vi "Offset_decoder_CH0_no_sign.vi"(11 "Array In1":i8[](array[numeric])) -> (3 "CH0":i32)   [LabVIEW 2012]
panel:
  out "CH0 3":u8 format="%x"
  out "CH0 2":u8 format="%x"
  out "CH0 1":u8 format="%x"
  out "CH0 0":u8 format="%x"
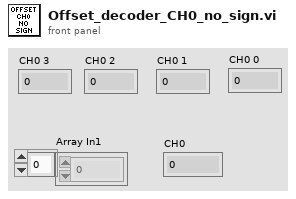
[diagram p1: front panel]
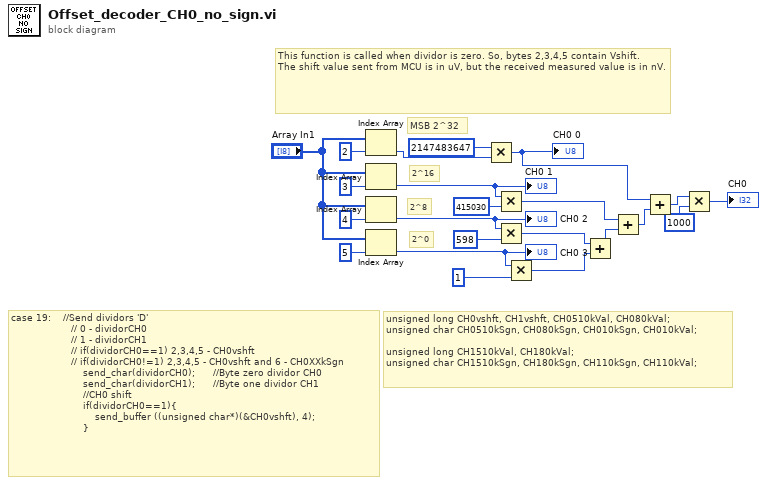
[diagram p0: block diagram]
diagram:
  # "2^0"
  # "2^8"
  # "2^16"
  # "MSB 2^32"
  # "unsigned long CH0vshft, CH1vshft, CH0510kVal, CH080kVal;\nunsigned char CH0510kSgn, CH080kSgn, CH010kSgn, CH010kVal;\n\nunsigned long CH1510kVal, CH180kVal;\nunsigned char CH1510kSgn, CH180kSgn, CH110kSgn, CH110kVal;"
  # "This function is called when dividor is zero. So, bytes 2,3,4,5 contain Vshift.\nThe shift value sent from MCU is in uV, but the received measured value is in nV."
  # "case 19:    //Send dividors 'D'\n                    // 0 - dividorCH0\n                    // 1 - dividorCH1\n                    // if(dividorCH0==1) 2,3,4,5 - CH0vshft\n                    // if(dividorCH0!=1) 2,3,4,5 - CH0vshft and 6 - CH0XXkSgn\n                        send_char(dividorCH0);      //Byte zero dividor CH0\n                        send_char(dividorCH1);      //Byte one dividor CH1\n                        //CH0 shift\n                        if(dividorCH0==1){\n                            send_buffer ((unsigned char*)(&CH0vshft), 4);\n                        }"
  n1 = Index Array(array="Array In1", index=2) -> (element=w5:i8)
  n2 = Index Array(array="Array In1", index=3) -> (element=w13:i8)
  "CH0 1" <- w13
  n3 = Index Array(array="Array In1", index=4) -> (element=w15:i8)
  "CH0 2" <- w15
  n4 = Index Array(array="Array In1", index=5) -> (element=w17:i8)
  "CH0 3" <- w17
  n5 = Multiply(x=2147483647, y=w5) -> (x*y=w6:i32)
  "CH0 0" <- w6
  n6 = Multiply(x=w13, y=415030) -> (x*y=w9:i32)
  n7 = Multiply(x=w15, y=598) -> (x*y=w12:i32)
  n8 = Multiply(x=w17, y=1) -> (x*y=w11:i32)
  n9 = Add(x=w12, y=w11) -> (x+y=w10:i32)
  n10 = Add(x=w9, y=w10) -> (x+y=w8:i32)
  n11 = Add(x=w6, y=w8) -> (x+y=w2:i32)
  n12 = Multiply(x=w2, y=1000) -> (x*y=→"CH0":i32)
